vi "send image reference.vi"(8 "error in (no error)":errorcluster, 11 "DAQOrcaFlash in":refnum<class "DAQOrcaFlash.lvclass">) -> (0 "error out":errorcluster, 3 "DAQOrcaFlash out":refnum<class "DAQOrcaFlash.lvclass">)   [LabVIEW 2012, in "DAQOrcaFlash.lvclass"]
uses:
  DAQOrcaFlash.lvclass
  DAQOrcaFlash.lvclass/DAQOrcaFlash.ctl
  <vilib>/Distrio/Murmex/Murmex/Murmex.lvclass
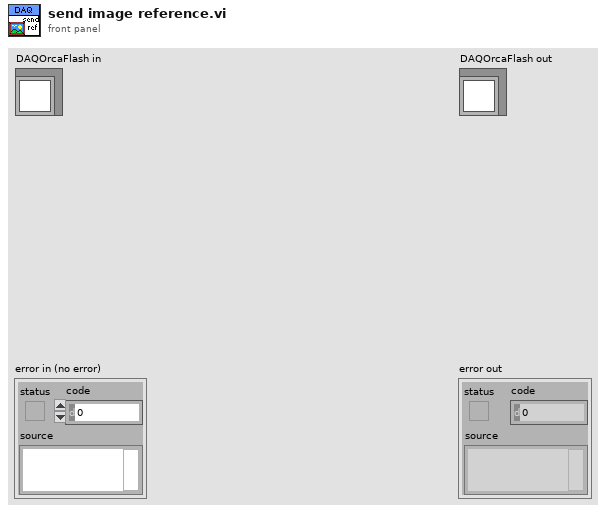
[diagram p1: front panel]
types:
  T1 = typedef "IMAQ Image.ctl" = refnum<image>
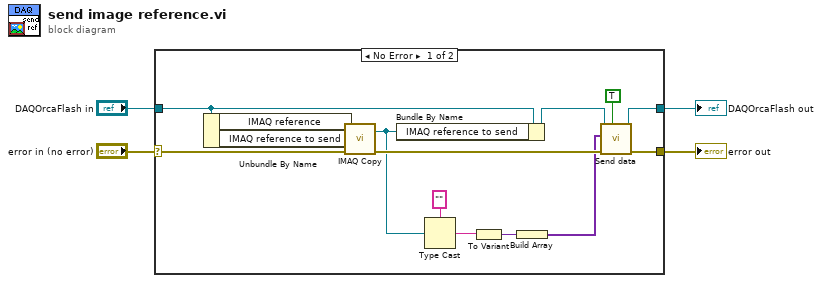
[diagram p0: block diagram]
diagram:
  n1 = case shown="No Error" "error in (no error)" {
    selector: "error in (no error)" -> [w16 w20]
    tunnel: [w12 w20] -> w3
    tunnel: [w10 w19] -> w1
    tunnel: "DAQOrcaFlash in" -> [w15 w19]
    frame No Error {
      n2 = Unbundle By Name(w15) -> ("IMAQ reference"=w18:T1, "IMAQ reference to send"=w17:T1)
      n3 = call "IMAQ Copy"("error in (no error)"=w16, "Image Dst"=w17, "Image Src"=w18) -> ("error out"=w13:errorcluster, "Image Dst Out"=w7:T1)  [unwired: 3 in]
      n4 = Bundle By Name(cluster=w15, "IMAQ reference to send"=w7) -> (w11:refnum<class "DAQOrcaFlash.lvclass">)
      n5 = Type Cast(type="", x=w7) -> (*(type *) &x=w5:string)
      n6 = To Variant(anything=w5) -> (Variant=w14:variant)
      n7 = Build Array(w14) -> (w9:variant[])
      n8 = call <vilib>:"Send data.vi"("is finalised data? (T)"=TRUE, "error in (no error)"=w13, "data (channels array)"=w9, "Murmex in"=w11) -> ("error out"=w12:errorcluster, "Murmex out"=w10:refnum<class "DAQOrcaFlash.lvclass">)  [unwired: 6 in]
    }
    frame Error {
    }
  }
  "error out" <- w3
  "DAQOrcaFlash out" <- w1
